vi "AudioStreamer.Get Status.vi"() -> (0 "status":string)   [LabVIEW 2020]
uses:
  Typedefs/AudioStreamer.Globals.vi
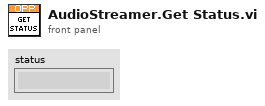
[diagram p1: front panel]
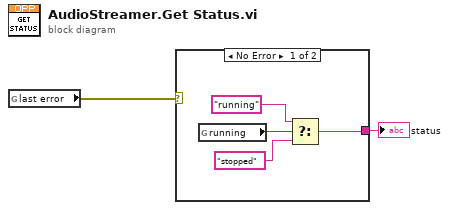
[diagram p0: block diagram]
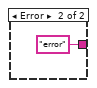
[diagram p2: hidden frame]
diagram:
  n1 = global read "AudioStreamer.Globals.vi" "last error"() -> (w2:errorcluster)
  n2 = case shown="No Error" w2 {
    tunnel: [w3 "error"] -> w1
    frame No Error {
      n3 = global read "AudioStreamer.Globals.vi" "running"() -> (w6:bool)
      n4 = Select(t="running", s=w6, f="stopped") -> (s? t:f=w3:string)
    }
    frame Error {
    }
  }
  "status" <- w1
